vi "20211001_HW01.vi"() -> ()   [LabVIEW 2019]
uses:
  <vilib>/Utility/miscctls.llb/LVBoundsTypeDef.ctl
panel:
  in  "Button":bool
  in  "Add.Btn.Size":bool
  in  "Add Button Size":T1={"Width"=10, "Height"=10}
  in  "Button Size":T1={"Width"=120, "Height"=120}
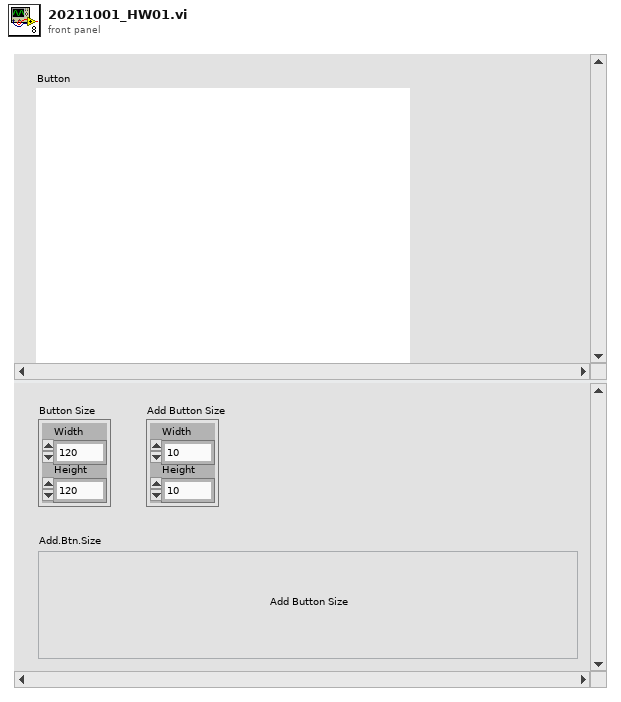
[diagram p1: front panel]
types:
  T1 = typedef "LVBoundsTypeDef.ctl" = cluster{"Width":u32, "Height":u32}
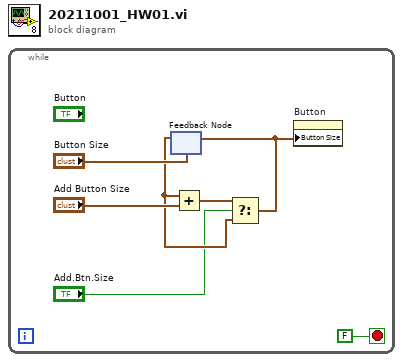
[diagram p0: block diagram]
diagram:
  n1 = while {
    stop <- FALSE stop-if-true
    n2 = feedback #1("Button Size") -> (w4:T1)
    n3 = Add(x=w4, y="Add Button Size") -> (x+y=w5:T1)
    n4 = Select(t=w5, s="Add.Btn.Size", f=w4) -> (s? t:f=w3:T1)
    n5 = feedback-in #1(w3) -> ()
    n6 = property on="Button" class="Bool (strict)"("Button Size"=w3) -> ()  [unwired: 2 in, 2 out]
  }
